vi "APP_Bit2Byte.vi"(11 "input bit stream":i8[](array[numeric])) -> (3 "output byte stream":u8[](array[numeric]))   [LabVIEW 2014]
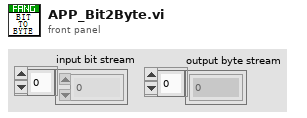
[diagram p1: front panel]
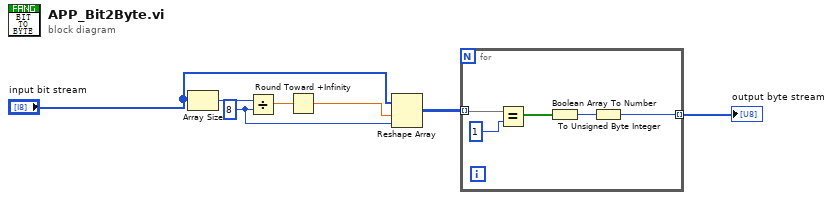
[diagram p0: block diagram]
diagram:
  w4 = 8 ("y")
  n1 = Array Size(array="input bit stream") -> (size(s)=w7:i32)
  n2 = Divide(x=w7, y=w4) -> (x/y=w6:dbl)
  n3 = Round Toward +Infinity(x=w6) -> (ceil(x): smallest int >= x=w5:dbl)
  n4 = Reshape Array("input bit stream", w5, w4) -> (w3:i8[][])
  n5 = for {
    tunnel: w3 -> [w12] mode=indexing
    tunnel: [w8] -> w1 mode=indexing
    n6 = Equal?(x=w12, y=1) -> (x = y?=w10:bool[])
    n7 = Boolean Array To Number(Boolean array=w10) -> (number=w9:u32)
    n8 = To Unsigned Byte Integer(number=w9) -> (unsigned 8bit integer=w8:u8)
  }
  "output byte stream" <- w1
